vi "Main Scan Processor Status.vi"() -> ()   [LabVIEW 2014]
panel:
  out "Busy":bool
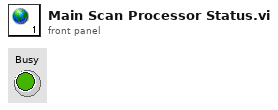
[diagram p1: front panel]
diagram:
